vi "AD.vi"(8 "error in (no error)":errorcluster, 10 "Canal":u8, 11 "Serial Devices in":refnum<class "Serial Devices.lvclass">) -> (0 "error out":errorcluster, 3 "Serial Devices out":refnum<class "Serial Devices.lvclass">)   [LabVIEW 2019, in "Serial Devices.lvlib" / "Serial Devices.lvclass"]
uses:
  Serial Devices.lvclass
  C:/Program Files (x86)/National Instruments/LabVIEW 2019/vi.lib/ActorFramework/Actor/Actor.lvclass
  Serial Devices.lvclass/Serial Devices.ctl
  <vilib>/ActorFramework/Actor/Actor.lvclass/Actor.ctl
  <vilib>/ActorFramework/Message Enqueuer/Message Enqueuer.lvclass/Message Enqueuer.ctl
  NXP/NXP.lvclass
  TI/CYPRESS.lvclass
  SIMULATED/SIMULATED.lvclass
  <vilib>/ActorFramework/Message Enqueuer/Init from Existing Queue.vi
  <vilib>/ActorFramework/Message Enqueuer/Message Enqueuer.lvclass
  <vilib>/ActorFramework/Actor/Actor.lvclass
  Serial Devices.lvlib
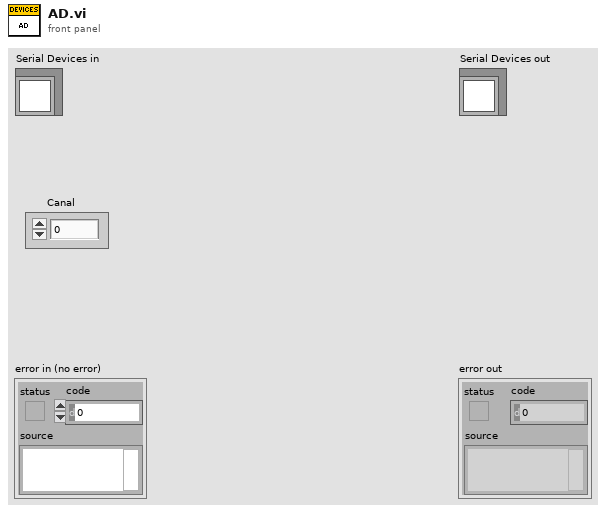
[diagram p1: front panel]
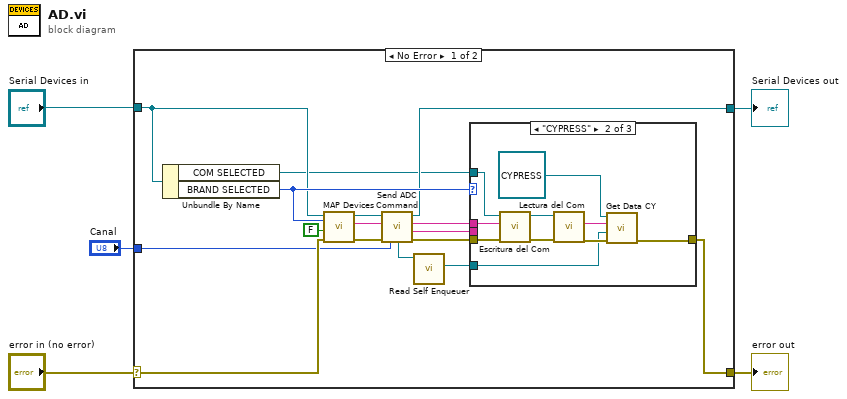
[diagram p0: block diagram]
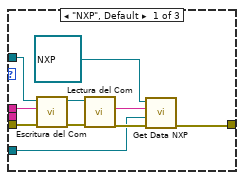
[diagram p2: hidden frame]
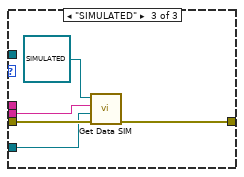
[diagram p3: hidden frame]
diagram:
  n1 = case shown="No Error" "error in (no error)" {
    selector: "error in (no error)" -> [w19 w47]
    tunnel: [w9 w47] -> w4
    tunnel: [w10 w46] -> w2
    tunnel: "Serial Devices in" -> [w8 w46]
    tunnel: "Canal" -> [w17 _]
    frame No Error {
      n2 = Unbundle By Name(w8) -> ("COM SELECTED"=w7:refnum<visa-resource-name>, "BRAND SELECTED"=w15:enum16{"NXP", "CYPRESS", "SIMULATED"})
      n3 = call "MAP Devices.vi"("error in (no error)"=w19, "CREAR"=FALSE, "BRAND SELECTED"=w15, "Serial Devices in"=w8) -> ("error out"=w16:errorcluster, "VALOR"=w18:string, "Serial Devices out"=w11:refnum<class "Serial Devices.lvclass">)  [unwired: 5 in]
      n4 = call-dynamic "Send ADC Command.vi"("error in"=w16, "Chanel"=w17, "Device"=w18, "Serial Devices in"=w11) -> ("error out"=w14:errorcluster, "Expected"=w13:string, "Command"=w6:string, "Serial Devices out"=w10:refnum<class "Serial Devices.lvclass">)  [unwired: 4 in]
      n5 = call <vilib>:"Read Self Enqueuer.vi"("Actor"=w11) -> ("Self Enqueuer"=w12:refnum<class "Message Enqueuer.lvclass">)  [unwired: 10 in]
      n6 = case shown="\"CYPRESS\"" w15 {
        tunnel: w14 -> [w30 w40 w44]
        tunnel: w13 -> [_ _ w43]
        tunnel: w12 -> [w22 w32 w42]
        tunnel: [w21 w31 w41] -> w9
        tunnel: w7 -> [w28 w39 _]
        tunnel: w6 -> [w29 w38 _]
        frame "NXP", Default {
          n7 = call "Escritura del Com.vi"("error in (no error)"=w30, "write buffer"=w29, "VISA Refnum in"=w28) -> ("error out"=w26:errorcluster, "VISA resource name out"=w27:refnum<visa-resource-name>)  [unwired: 7 in]
          n8 = call "Lectura del Com.vi"("error in (no error)"=w26, "VISA Refnum in"=w27) -> ("error out"=w23:errorcluster, "Serial Response"=w24:string)  [unwired: 7 in, 1 out]
          n9 = call "Get Data NXP.vi"("error in"=w23, "Data Enqueuer"=w22, "Data"=w24, "NXP in"=refnum<class "NXP.lvclass"> refnum ("NXP.lvclass")) -> ("error out"=w21:errorcluster)  [unwired: 6 in, 1 out]
        }
        frame "CYPRESS" {
          n10 = call "Escritura del Com.vi"("error in (no error)"=w40, "write buffer"=w38, "VISA Refnum in"=w39) -> ("error out"=w37:errorcluster, "VISA resource name out"=w36:refnum<visa-resource-name>)  [unwired: 7 in]
          n11 = call "Lectura del Com.vi"("error in (no error)"=w37, "VISA Refnum in"=w36) -> ("error out"=w33:errorcluster, "Serial Response"=w34:string)  [unwired: 7 in, 1 out]
          n12 = call "Get Data CY.vi"("error in"=w33, "Data Enqueuer"=w32, "Data"=w34, "CYPRESS in"=refnum<class "CYPRESS.lvclass"> refnum ("CYPRESS.lvclass")) -> ("error out"=w31:errorcluster)  [unwired: 6 in, 1 out]
        }
        frame "SIMULATED" {
          n13 = call "Get Data SIM.vi"("error in"=w44, "Data Enqueuer"=w42, "Data"=w43, "SIMULATED in"=refnum<class "SIMULATED.lvclass"> refnum ("SIMULATED.lvclass")) -> ("error out"=w41:errorcluster)  [unwired: 6 in, 1 out]
        }
      }
    }
    frame Error {
    }
  }
  "error out" <- w4
  "Serial Devices out" <- w2
